vi "主通讯程序.vi"   [LabVIEW 2012]
uses:
  <vilib>/Instr/_visa.llb/VISA Configure Serial Port (Instr).vi
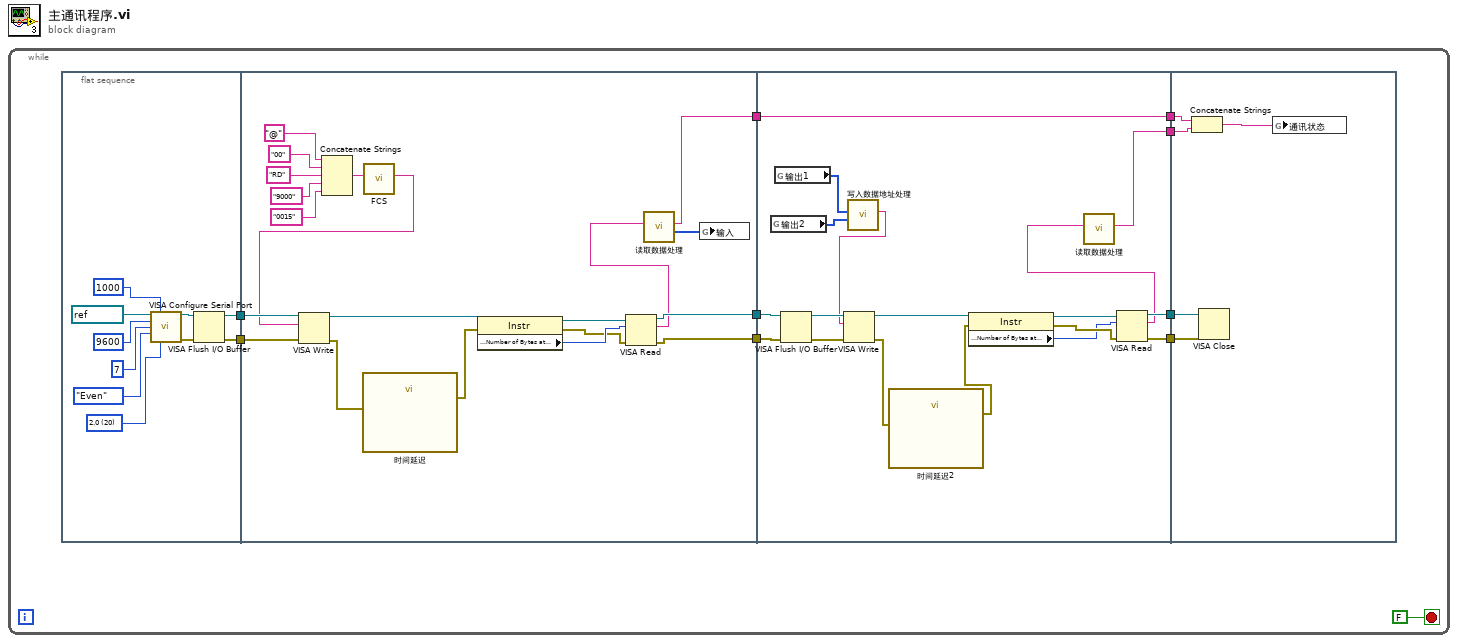
[diagram p0: block diagram]
diagram:
  n1 = while {
    stop <- FALSE stop-if-true
    n2 = flat-sequence {
      tunnel: [w13] -> w10
      tunnel: [w11] -> w9
      tunnel: w10 -> [w40]
      tunnel: w9 -> [w39]
      tunnel: [w34] -> w8
      tunnel: [w33] -> w7
      tunnel: [w21] -> w6
      tunnel: w8 -> [w58]
      tunnel: w7 -> [w57]
      tunnel: [w50] -> w5
      tunnel: [w49] -> w4
      tunnel: [w42] -> w3
      tunnel: w6 -> [w42]
      tunnel: [w41] -> w2
      tunnel: w5 -> [w63]
      tunnel: w4 -> [w62]
      tunnel: w3 -> [w61]
      tunnel: w2 -> [w60]
      frame #0 {
        w15 = u16 20 items=["1.0"=10, "1.5"=15, "2.0"=20] ("stop bits (10: 1 bit)")
        n3 = call-poly "VISA Configure Serial Port"("VISA resource name"=refnum<visa-resource-name> "COM2", "timeout (10sec)"=u32 1000, "baud rate (9600)"=u32 9600, "data bits (8)"=u16 7, "parity (0:none)"=enum16{"None", "Odd", "Even", "Mark", "Space"}."Even", "stop bits (10: 1 bit)"=w15) -> ("VISA resource name out"=w14:refnum<visa-resource-name>, "error out"=w12:errorcluster)  [unwired: 8 in]
        n4 = VISA Flush I/O Buffer(VISA resource name=w14, error in (no error)=w12) -> (VISA resource name out=w13:refnum<visa-resource-name>, error out=w11:errorcluster)  [unwired: 1 in]
      }
      frame #1 {
        n5 = Concatenate Strings("@" ("字符串"), "00" ("字符串"), "RD" ("字符串"), "9000" ("字符串"), "0015" ("字符串")) -> (w25:string)
        n6 = call "FCS.vi"("发送命令"=w25) -> ("完整帧"=w24:string)  [unwired: 9 in, 1 out]
        n7 = VISA Write(VISA resource name=w40, write buffer=w24, error in (no error)=w39) -> (VISA resource name out=w38:refnum<visa-resource-name>, error out=w32:errorcluster)  [unwired: 1 out]
        n8 = call "时间延迟"("error in (no error)"=w32) -> ("error out"=w31:errorcluster)  [unwired: 10 in]
        n9 = property class="Instr"(reference=w38, error in=w31) -> (reference out=w37:refnum<visa-resource-name>, error out=w35:errorcluster, "Serial Settings:Number of Bytes at Serial Port"=w36:u32)
        n10 = VISA Read(VISA resource name=w37, byte count=w36, error in (no error)=w35) -> (VISA resource name out=w34:refnum<visa-resource-name>, read buffer=w23:string, error out=w33:errorcluster)  [unwired: 1 out]
        n11 = call "读取数据处理.vi"("通讯读取数据"=w23) -> ("读取数据"=w22:i16[], "通讯状态"=w21:string)  [unwired: 9 in]
        n12 = global write "通讯数据.vi" "输入"(w22) -> ()
      }
      frame #2 {
        n13 = global read "通讯数据.vi" "输出2"() -> (w45:u16[])
        n14 = global read "通讯数据.vi" "输出1"() -> (w46:u16[])
        n15 = VISA Flush I/O Buffer(VISA resource name=w58, error in (no error)=w57) -> (VISA resource name out=w52:refnum<visa-resource-name>, error out=w51:errorcluster)  [unwired: 1 in]
        n16 = call "写入数据地址处理.vi"("输入2"=w45, "输入1"=w46) -> ("完整帧"=w44:string)  [unwired: 9 in]
        n17 = VISA Write(VISA resource name=w52, write buffer=w44, error in (no error)=w51) -> (VISA resource name out=w53:refnum<visa-resource-name>, error out=w47:errorcluster)  [unwired: 1 out]
        n18 = call "时间延迟2"("error in (no error)"=w47) -> ("error out"=w48:errorcluster)  [unwired: 10 in]
        n19 = property class="Instr"(reference=w53, error in=w48) -> (reference out=w54:refnum<visa-resource-name>, error out=w56:errorcluster, "Serial Settings:Number of Bytes at Serial Port"=w55:u32)
        n20 = VISA Read(VISA resource name=w54, byte count=w55, error in (no error)=w56) -> (VISA resource name out=w50:refnum<visa-resource-name>, read buffer=w43:string, error out=w49:errorcluster)  [unwired: 1 out]
        n21 = call "读取数据处理.vi"("通讯读取数据"=w43) -> ("通讯状态"=w41:string)  [unwired: 9 in, 1 out]
      }
      frame #3 {
        n22 = Concatenate Strings(w61, w60) -> (w59:string)
        n23 = VISA Close(VISA resource name=w63, error in (no error)=w62) -> ()  [unwired: 1 out]
        n24 = global write "通讯数据.vi" "通讯状态"(w59) -> ()
      }
    }
  }
